vi "Load Data Types.vi"(8 "error in (no error)":errorcluster) -> (0 "error out":errorcluster, 2 "Data Type Names":string[](array[string]), 3 "Data Type Objects":refnum<class "Generic Data Type.lvclass">[](array[class]))   [LabVIEW 2018, in "Generic Data Type.lvclass"]
uses:
  Generic Data Type.lvclass
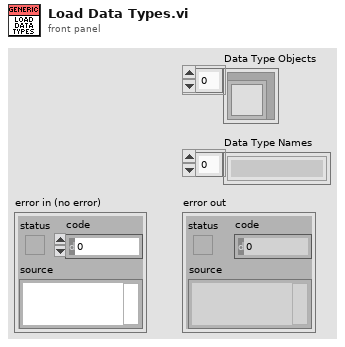
[diagram p1: front panel]
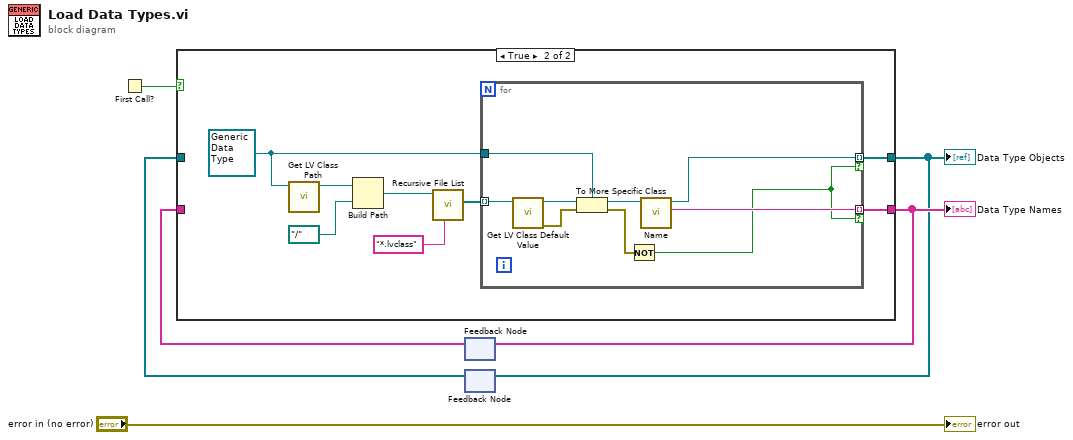
[diagram p0: block diagram]
diagram:
  n1 = First Call?() -> (First Call?: T/F=w5:bool)
  n2 = feedback #1() -> (w3:string[])  [unwired: 1 in]
  n3 = feedback #2() -> (w1:refnum<class "Generic Data Type.lvclass">[])  [unwired: 1 in]
  n4 = case shown="True" w5 {
    tunnel: [w8 w10] -> w4
    tunnel: w3 -> [w8 _]
    tunnel: [w7 w9] -> w2
    tunnel: w1 -> [w7 _]
    frame False {
    }
    frame True {
      w11 = refnum<class "Generic Data Type.lvclass"> refnum ("Generic Data Type")
      n5 = call <vilib>:"Get LV Class Path.vi"("object"=w11) -> ("class path"=w16:path)  [unwired: 9 in, 1 out]
      n6 = Build Path(base path=w16, name or relative path=path "../..") -> (appended path=w14:path)
      n7 = call <vilib>:"Recursive File List.vi"("pattern"="*.lvclass", "Folder Path"=w14) -> ("All Files in Dir"=w12:path[])  [unwired: 5 in, 4 out]
      n8 = for {
        tunnel: w12 -> [w25] mode=indexing
        tunnel: w11 -> [w23]
        tunnel: [w18] -> w10 mode=indexing if=w17
        tunnel: [w21] -> w9 mode=indexing if=w17
        n9 = call <vilib>:"Get LV Class Default Value.vi"("class path"=w25) -> ("error out"=w19:errorcluster, "object"=w24:refnum<class>)  [unwired: 9 in]
        n10 = To More Specific Class(target class=w23, reference=w24, error in=w19) -> (specific class reference=w22:refnum<class "Generic Data Type.lvclass">, error out=w20:errorcluster)
        n11 = Not(x=w20) -> (.not. x?=w17:bool)
        n12 = call-dynamic "Name.vi"("Generic Data Type in"=w22) -> ("String"=w18:string, "Generic Data Type (dup)"=w21:refnum<class "Generic Data Type.lvclass">)  [unwired: 9 in]
      }
    }
  }
  "Data Type Names" <- w4
  "Data Type Objects" <- w2
  n13 = feedback-in #1(w4) -> ()
  n14 = feedback-in #2(w2) -> ()
  "error out" <- "error in (no error)"
